vi "subGetAllNodeAttributes.vi"(8 "error in (no error)":errorcluster, 11 "Node Reg in":refnum<k20>) -> (0 "error out":errorcluster, 1 "Attributes":map{string, string}(c390), 3 "Node Reg":refnum<k20>)   [LabVIEW 2020, in "DefaultExtensions.lvlib" / "CDefaultRuleFileParser.lvclass"]
uses:
  CDefaultRuleFileParser.lvclass
  <resource>/objmgr/DOMUserDefRef.rc
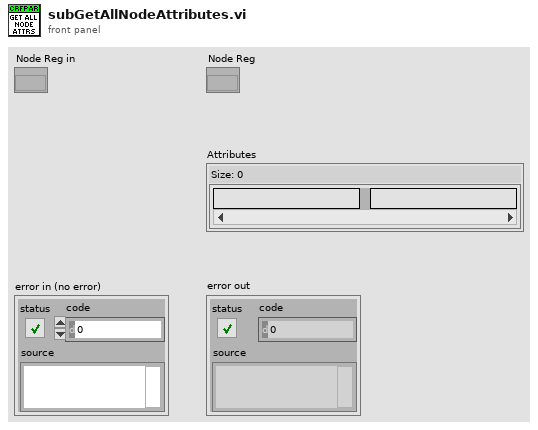
[diagram p1: front panel]
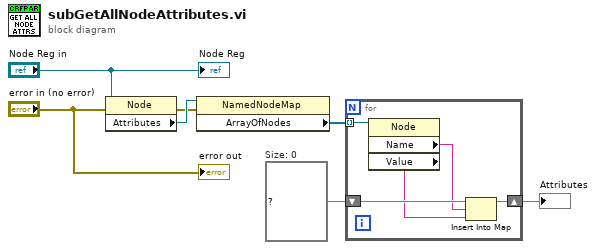
[diagram p0: block diagram]
diagram:
  w4 = map{string, string} {}  # Size: 0
  n1 = property class="Node"(reference="Node Reg in", error in="error in (no error)") -> (error out=w5:errorcluster, "Attributes"=w7:refnum<k20>)  [unwired: 1 out]
  n2 = property class="NamedNodeMap"(reference=w7, error in=w5) -> ("ArrayOfNodes"=w6:refnum<k20>[])  [unwired: 2 out]
  n3 = for {
    tunnel: w6 -> [w12] mode=indexing
    shift-right: [w8] -> w3
    shift-left: w4 -> [w11]
    n4 = property class="Node"(reference=w12) -> ("Name"=w10:string, "Value"=w9:string)  [unwired: 1 in, 2 out]
    n5 = Insert Into Map(map in=w11, key=w10, value=w9) -> (map out=w8:map{string, string})  [unwired: 2 out]
  }
  "Attributes" <- w3
  "Node Reg" <- "Node Reg in"
  "error out" <- "error in (no error)"
